vi "liftingCellMovement_v01.vi"(0 "manp in":T2={"Actuator COM"="COM6", "Actuator type"=enum."Scientifica"}, 1 "reset motion":T1=enum."slow", 5 "Current Position":i32[](array[numeric]), 7 "NumberOfIncrements":i32, 9 "Final Distance (steps)":i32, 11 "error in":errorcluster, 12 "NumberOfSpirals":i32) -> (4 "manip out":T2={"Actuator COM"="COM14", "Actuator type"=enum."Scientifica"}, 15 "error out":errorcluster)   [LabVIEW 2019]
uses:
  pipette cleaning/pressure box/cleaning_soft/controls/actuator_cluster.ctl
  pipette cleaning/pressure box/cleaning_soft/controls/actuator_type.ctl
  controls/scope_motion.ctl
panel:
  out "positionSequence":i32[][](array[numeric])
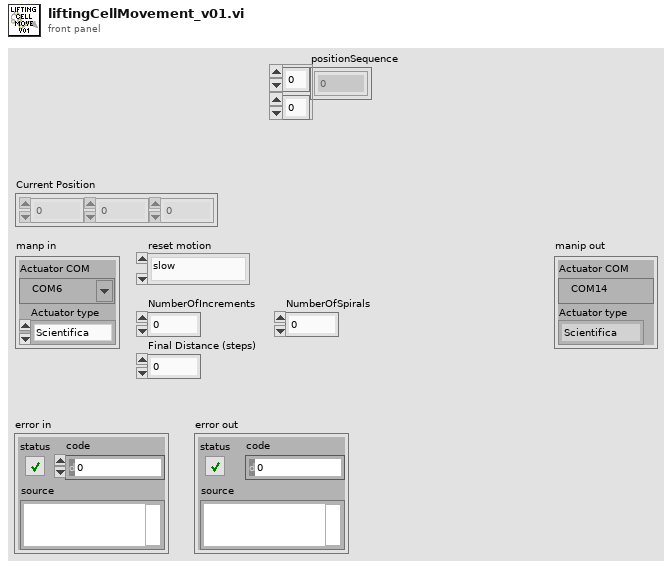
[diagram p1: front panel]
types:
  T1 = typedef "scope_motion.ctl" = enum16{"superSlow", "fast", "slow", "find slice speed", "slow_dualPatch"}
  T2 = typedef "actuator_cluster.ctl" = cluster{"Actuator COM":refnum<visa-resource-name>, "Actuator type":T3}
  T3 = typedef "actuator_type.ctl" = enum16{"Scientifica", "Sutter", "Demo", "Off"}
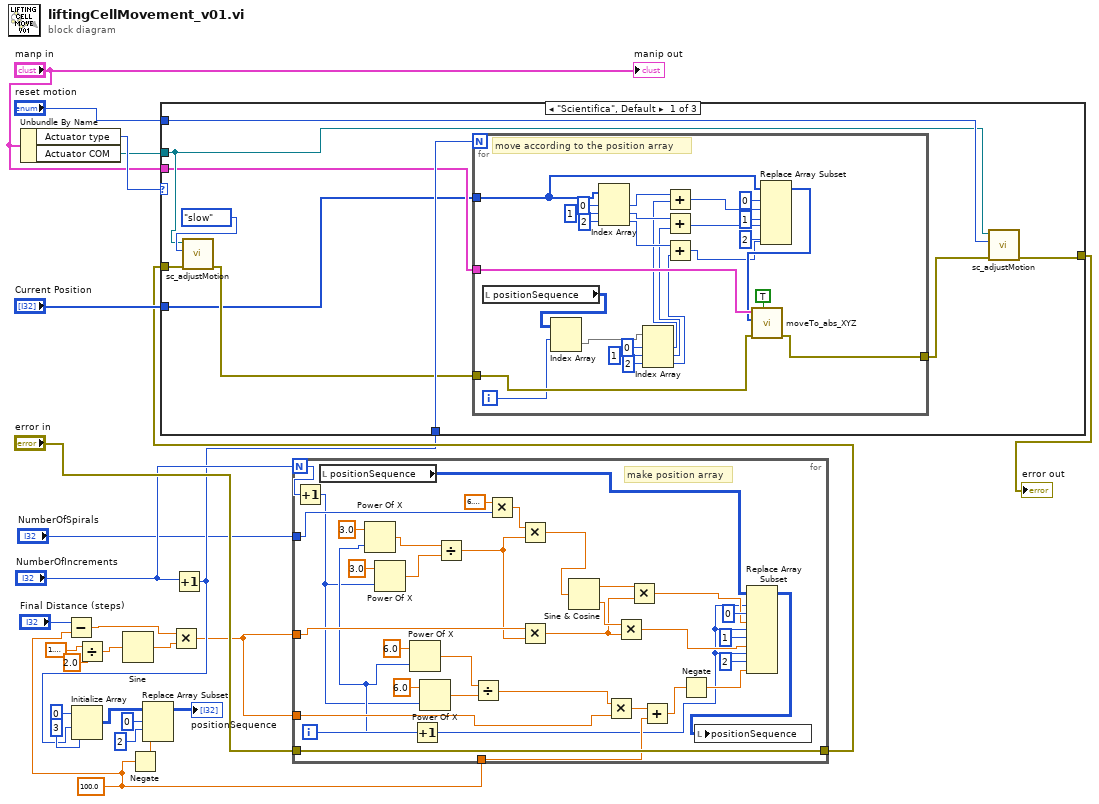
[diagram p0: block diagram]
diagram:
  w2 = 100.0 ("new element/subarray")
  n1 = Unbundle By Name("manp in") -> ("Actuator type"=w26:T3, "Actuator COM"=w25:refnum<visa-resource-name>)
  n2 = Subtract(x="Final Distance (steps)", y=w2) -> (x-y=w1:dbl)
  n3 = Divide(x=1.5707963267948966, y=2.0) -> (x/y=w13:dbl)
  n4 = Sine(x=w13) -> (sin(x)=w15:dbl)
  n5 = Negate(x=w2) -> (-x=w5:dbl)
  n6 = Multiply(x=w1, y=w15) -> (x*y=w7:dbl)
  n7 = Increment(x="NumberOfIncrements") -> (x+1=w9:i32)
  n8 = Initialize Array(0 ("element"), w9, 3 ("dimension size")) -> (w20:i32[][])
  n9 = Replace Array Subset(array=w20, new element=w5, index (row)=0 ("index"), index (col)=2 ("disabled index (col)")) -> (→"positionSequence":i32[][])
  n10 = for {
    N: "NumberOfIncrements" -> [w43]
    tunnel: w7 -> [w58]
    tunnel: "error in" -> [w56]
    tunnel: [w56] -> w11
    tunnel: "NumberOfSpirals" -> [w53]
    tunnel: w7 -> [w40]
    tunnel: w2 -> [w46]
    i -> [w42]
    # "make position array"
    n11 = Increment(x=w43) -> (x+1=w28:i32)
    n12 = local read "positionSequence"() -> (w55:i32[][])
    n13 = Power Of X(1:w28, 2:3.0 ("y")) -> (0:w33:dbl)
    n14 = Increment(x=w42) -> (x+1=w30:i32)
    n15 = Power Of X(1:w30, 2:3.0 ("y")) -> (0:w35:dbl)
    n16 = Power Of X(1:w30, 2:6.0 ("y")) -> (0:w29:dbl)
    n17 = Power Of X(1:w28, 2:6.0 ("y")) -> (0:w27:dbl)
    n18 = Divide(x=w35, y=w33) -> (x/y=w39:dbl)
    n19 = Divide(x=w29, y=w27) -> (x/y=w59:dbl)
    n20 = Multiply(x=6.283185307179586, y=w53) -> (x*y=w52:dbl)
    n21 = Multiply(x=w52, y=w39) -> (x*y=w49:dbl)
    n22 = Multiply(x=w40, y=w39) -> (x*y=w38:dbl)
    n23 = Sine & Cosine(0:w49) -> (1:w48:dbl, 2:w47:dbl)
    n24 = Multiply(x=w59, y=w58) -> (x*y=w41:dbl)
    n25 = Multiply(x=w47, y=w38) -> (x*y=w50:dbl)
    n26 = Multiply(x=w48, y=w38) -> (x*y=w51:dbl)
    n27 = Add(x=w41, y=w46) -> (x+y=w44:dbl)
    n28 = Negate(x=w44) -> (-x=w37:dbl)
    n29 = Replace Array Subset(array=w55, new element #1=w51, index (row) #1=w30, index (col) #1=0 ("index (row)"), new element #2=w50, index (row) #2=w30, index (col) #2=1 ("disabled index (col)"), new element #3=w37, index (row) #3=w30, index (col) #3=2 ("disabled index (col)")) -> (w57:i32[][])
    n30 = local write "positionSequence"(w57) -> ()
  }
  n31 = case shown="\"Scientifica\", Default" w26 {
    tunnel: w25 -> [w67 _ _]
    tunnel: w11 -> [w71 w99 w100]
    tunnel: [w68 w99 w100] -> w23
    tunnel: "reset motion" -> [w70 _ _]
    tunnel: w9 -> [w66 _ _]
    tunnel: "Current Position" -> [w62 _ _]
    tunnel: "manp in" -> [w65 _ _]
    frame "Scientifica", Default {
      n32 = call "sc_adjustMotion.vi"("error in (no error)"=w71, "motion"=scope_motion."slow", "VISA handle"=w67) -> ("error out"=w64:errorcluster)  [unwired: 7 in, 1 out]
      n33 = for {
        N: w66 -> [_]
        tunnel: w65 -> [w98]
        tunnel: w64 -> [w96]
        tunnel: [w95] -> w63
        tunnel: w62 -> [w83]
        i -> [w85]
        # "move according to the position array"
        n34 = local read "positionSequence"() -> (w72:i32[][])
        n35 = Index Array(array=w72, index (row)=w85) -> (element=w79:i32[])  [unwired: 1 in]
        n36 = Index Array(array=w83, index #1=0 ("index"), index #2=1 ("index"), index #3=2 ("index")) -> (element #1=w88:i32, element #2=w87:i32, element #3=w86:i32)
        n37 = Index Array(array=w79, index #1=0 ("index"), index #2=1 ("index"), index #3=2 ("index")) -> (element #1=w76:i32, element #2=w78:i32, element #3=w77:i32)
        n38 = Add(x=w88, y=w76) -> (x+y=w73:i32)
        n39 = Add(x=w87, y=w78) -> (x+y=w74:i32)
        n40 = Add(x=w86, y=w77) -> (x+y=w75:i32)
        n41 = Replace Array Subset(array=w83, new element #1=w73, index #1=0 ("index"), new element #2=w74, index #2=1 ("index"), new element #3=w75, index #3=2 ("index")) -> (w84:i32[])
        n42 = call "moveTo_abs_XYZ.vi"("blocking?"=TRUE, "error in"=w96, "XYZ location (steps)"=w84, "Actuator cluster in"=w98) -> ("error out"=w95:errorcluster)  [unwired: 6 in, 1 out]
      }
      n43 = call "sc_adjustMotion.vi"("error in (no error)"=w63, "motion"=w70, "VISA handle"=w67) -> ("error out"=w68:errorcluster)  [unwired: 7 in, 1 out]
    }
    frame "Sutter" {
    }
    frame "Demo" {
    }
  }
  "error out" <- w23
  "manip out" <- "manp in"
